vi "Encode Message.vi"(8 "Error In":errorcluster, 10 "Message In":string, 11 "Image 1 Path in":path) -> (0 "Error Out":errorcluster, 3 "Image 2 Path out":path)   [LabVIEW 2020]
uses:
  SubVIs/Compression Type.ctl
  SubVIs/Encode Byte.vi
  SubVIs/Header Size.vi
  SubVIs/Encode I32.vi
  Image Comparison/Image Comparison.lvclass
panel:
  out "Bytes Free":i32
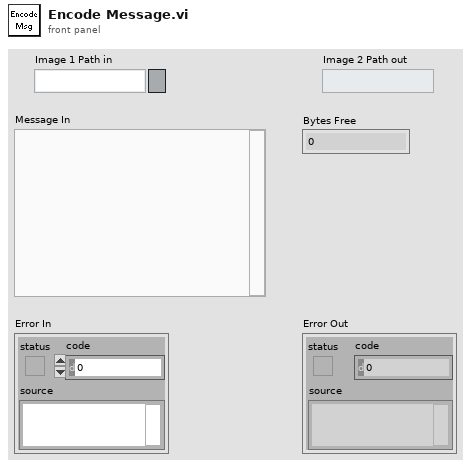
[diagram p1: front panel]
types:
  T1 = typedef "Compression Type.ctl" = enum8{"zip", "7z", "zpaq"}
  T2 = typedef "imagedata.ctl" = cluster{"image type":i32, "image depth":i32, "image":u8[], "mask":u8[], "colors":u32[], "Rectangle":cluster{"left":i16, "top":i16, "right":i16, "bottom":i16}}
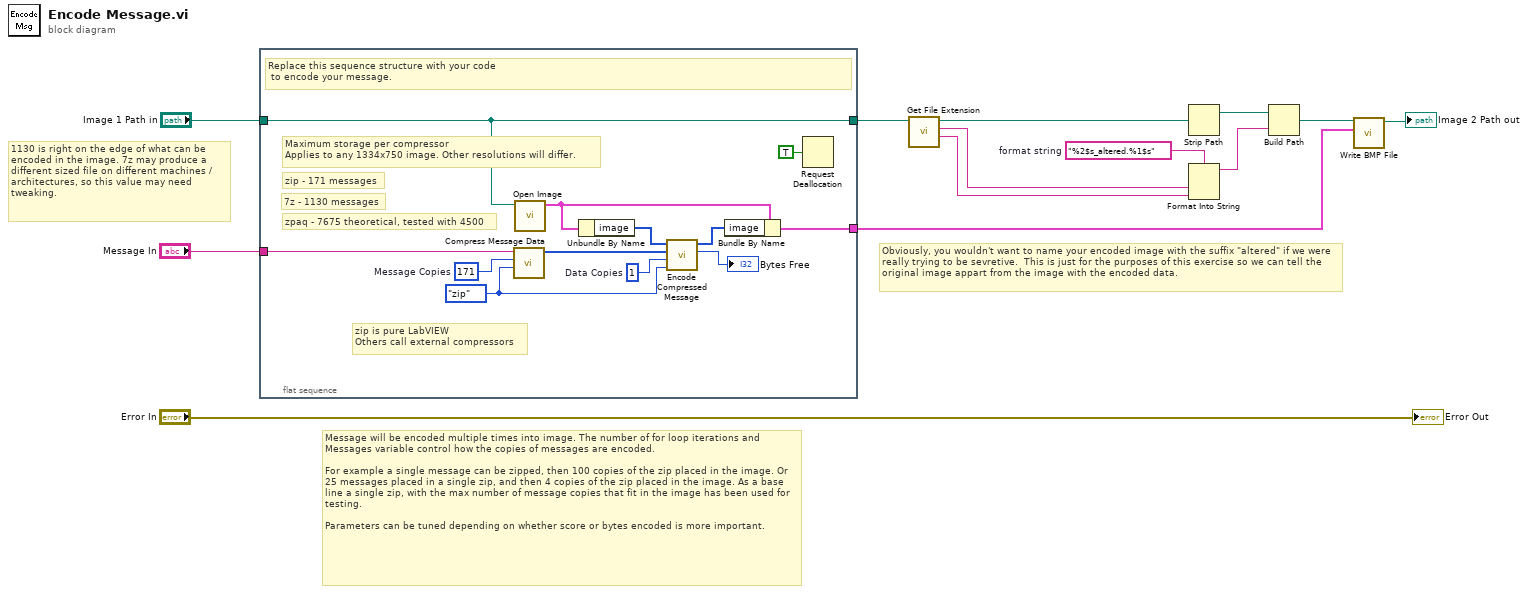
[diagram p0: block diagram]
diagram:
  w8 = "%2$s_altered.%1$s"  # format string
  # "1130 is right on the edge of what can be encoded in the image. 7z may produce a different sized file on different machines / architectures, so this value may need tweaking."
  # "Message will be encoded multiple times into image. The number of for loop iterations and Messages variable control how the copies of messages are encoded.\n\nFor example a single message can be zipped, then 100 copies of the zip placed in the image. Or 25 messages placed in a single zip, and then 4 copies of the zip placed in the image. As a base line a single zip, with the max number of message copies that fit in the image has been used for testing.\n\nParameters can be tuned depending on whether score or bytes encoded is more important."
  # "Obviously, you wouldn't want to name your encoded image with the suffix \"altered\" if we were really trying to be sevretive.  This is just for the purposes of this exercise so we can tell the original image appart from the image with the encoded data."
  n1 = flat-sequence {
    tunnel: "Message In" -> [w15]
    tunnel: "Image 1 Path in" -> [w20]
    tunnel: [w20] -> w10
    tunnel: [w22] -> w1
    frame #0 {
      w16 = Compression_Type."zip" ("Compression (zip)")
      w21 = 1  # Data Copies
      w14 = 171  # Message Copies
      # "Maximum storage per compressor\nApplies to any 1334x750 image. Other resolutions will differ."
      # "zpaq - 7675 theoretical, tested with 4500"
      # "zip is pure LabVIEW\nOthers call external compressors"
      # "7z - 1130 messages"
      # "zip - 171 messages"
      # "Replace this sequence structure with your code\n to encode your message."
      n2 = call "Compress Message Data.vi"("Compression (zip)"=w16, "Copies (1)"=w14, "Message"=w15) -> ("Compressed Message"=w25:u8[])  [unwired: 8 in]
      n3 = call "Open Image.vi"("Image"=w20) -> ("image data"=w19:T2)  [unwired: 9 in, 1 out]
      n4 = Unbundle By Name(w19) -> ("image"=w24:u8[])
      n5 = call "Encode Compressed Message.vi"("Compression (zip)"=w16, "Messages to Encode (-1)"=w21, "Array To Encode"=w25, "Image In"=w24) -> ("Bytes Free"=→"Bytes Free":i32, "Image Out"=w23:u8[])  [unwired: 6 in]
      n6 = Bundle By Name(cluster=w19, "image"=w23) -> (w22:T2)
      n7 = Request Deallocation(TRUE ("flag")) -> ()
    }
  }
  n8 = call <vilib>:"Get File Extension.vi"("file"=w10) -> ("filename without extension"=w5:string, "lowercase file extension"=w4:string, "dup file"=w9:path)  [unwired: 6 in, 2 out]
  n9 = Strip Path(path=w9) -> (stripped path=w7:path)  [unwired: 1 out]
  n10 = Format Into String(format string=w8, w4, w5) -> (resulting string=w6:string)  [unwired: 2 in, 1 out]
  n11 = Build Path(base path=w7, name or relative path=w6) -> (appended path=w3:path)
  n12 = call <vilib>:"Write BMP File.vi"("image data"=w1, "path to BMP file"=w3) -> ("path"=→"Image 2 Path out":path)  [unwired: 8 in, 1 out]
  "Error Out" <- "Error In"
